vi "Order JointCommands By Name.vi"(0 "Ordered Joint Names":string[](array[string]), 2 "JointCommands":T1) -> (7 "Ordered JointCommands":T1)   [LabVIEW 2013]
uses:
  Grips Robot/JointCommands.ctl
  Grips Robot/Grips Robot.lvclass
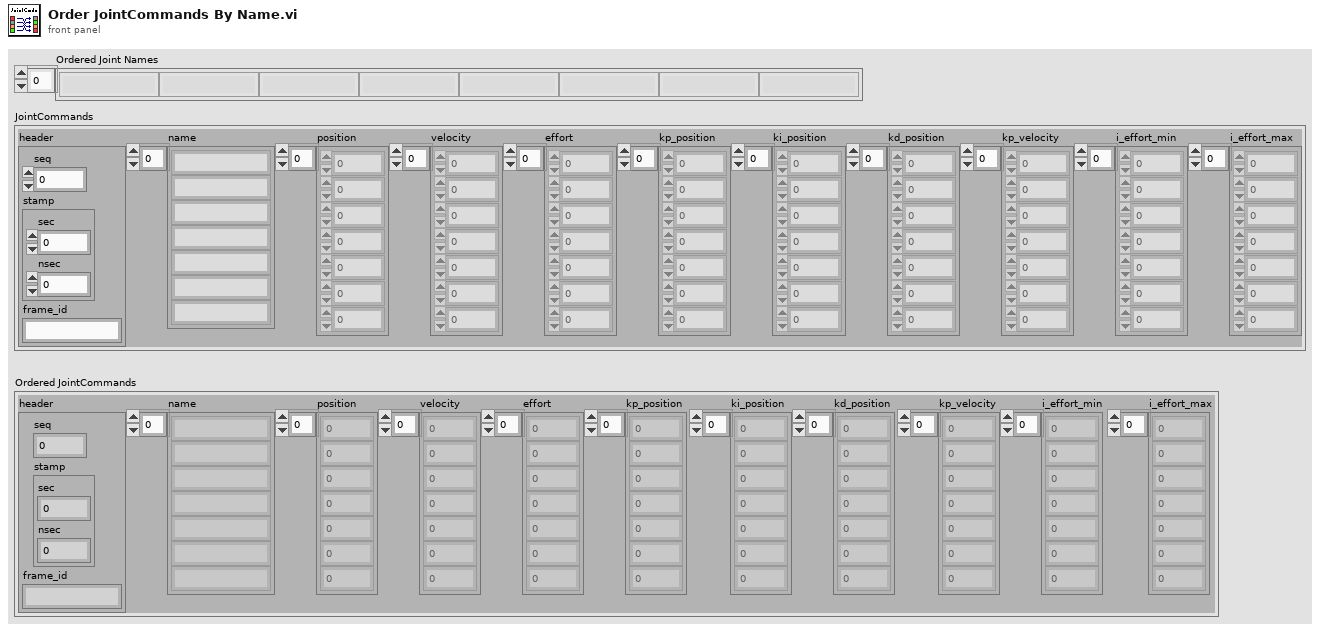
[diagram p1: front panel]
types:
  T1 = typedef "Grips Robot.lvclass/JointCommands.ctl" = cluster{"header":cluster{"seq":u32, "stamp":cluster{"sec":i32, "nsec":i32}, "frame_id":string}, "name":string[], "position":dbl[], "velocity":dbl[], "effort":dbl[], "kp_position":dbl[], "ki_position":dbl[], "kd_position":dbl[], "kp_velocity":dbl[], "i_effort_min":dbl[], "i_effort_max":dbl[]}
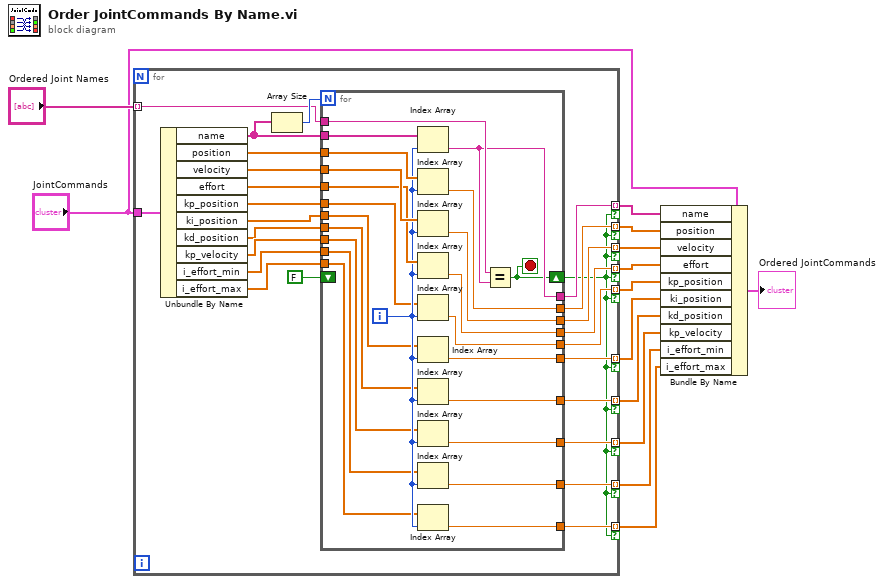
[diagram p0: block diagram]
diagram:
  n1 = for {
    tunnel: "JointCommands" -> [w38]
    tunnel: "Ordered Joint Names" -> [w35] mode=indexing
    tunnel: [w24] -> w10 mode=indexing if=w14
    tunnel: [w23] -> w9 mode=indexing if=w14
    tunnel: [w22] -> w8 mode=indexing if=w14
    tunnel: [w21] -> w7 mode=indexing if=w14
    tunnel: [w20] -> w6 mode=indexing if=w14
    tunnel: [w19] -> w5 mode=indexing if=w14
    tunnel: [w18] -> w4 mode=indexing if=w14
    tunnel: [w17] -> w3 mode=indexing if=w14
    tunnel: [w16] -> w2 mode=indexing if=w14
    tunnel: [w15] -> w1 mode=indexing if=w14
    n2 = Unbundle By Name(w38) -> ("name"=w36:string[], "position"=w34:dbl[], "velocity"=w33:dbl[], "effort"=w32:dbl[], "kp_position"=w25:dbl[], "ki_position"=w26:dbl[], "kd_position"=w27:dbl[], "kp_velocity"=w28:dbl[], "i_effort_min"=w29:dbl[], "i_effort_max"=w30:dbl[])
    n3 = Array Size(array=w36) -> (size(s)=w37:i32)
    n4 = for {
      N: w37 -> [_]
      tunnel: w36 -> [w61]
      tunnel: w35 -> [w60]
      tunnel: w34 -> [w59]
      tunnel: w33 -> [w58]
      tunnel: w32 -> [w57]
      tunnel: [w56] -> w15
      tunnel: [w55] -> w24
      tunnel: [w54] -> w23
      tunnel: [w53] -> w22
      shift-right: [w52] -> w14
      shift-left: FALSE -> [_]
      tunnel: w30 -> [w50]
      tunnel: w29 -> [w49]
      tunnel: w28 -> [w48]
      tunnel: w27 -> [w47]
      tunnel: w26 -> [w46]
      tunnel: w25 -> [w45]
      tunnel: [w44] -> w21
      tunnel: [w43] -> w20
      tunnel: [w42] -> w19
      tunnel: [w41] -> w18
      tunnel: [w40] -> w17
      tunnel: [w39] -> w16
      i -> [w51]
      stop <- w52 stop-if-true
      n5 = Index Array(array=w61, index=w51) -> (element=w56:string)
      n6 = Index Array(array=w59, index=w51) -> (element=w55:dbl)
      n7 = Index Array(array=w58, index=w51) -> (element=w54:dbl)
      n8 = Index Array(array=w57, index=w51) -> (element=w53:dbl)
      n9 = Index Array(array=w45, index=w51) -> (element=w44:dbl)
      n10 = Index Array(array=w46, index=w51) -> (element=w43:dbl)
      n11 = Index Array(array=w47, index=w51) -> (element=w42:dbl)
      n12 = Index Array(array=w48, index=w51) -> (element=w41:dbl)
      n13 = Index Array(array=w49, index=w51) -> (element=w40:dbl)
      n14 = Index Array(array=w50, index=w51) -> (element=w39:dbl)
      n15 = Equal?(x=w60, y=w56) -> (x = y?=w52:bool)
    }
  }
  n16 = Bundle By Name(cluster="JointCommands", "name"=w1, "position"=w10, "velocity"=w9, "effort"=w8, "kp_position"=w7, "ki_position"=w6, "kd_position"=w5, "kp_velocity"=w4, "i_effort_min"=w3, "i_effort_max"=w2) -> (→"Ordered JointCommands":T1)
